vi "Telescope GUI.vi"(9 "Standalone":bool=TRUE, 10 "Init Data":variant, 11 "Telescope Name":string) -> ()   [LabVIEW 2024]
uses:
  typedefs/CC enum Operation Mode.ctl
  Telescope cluster Settings.ctl
  CC cluster Telescope Offsets.ctl
  Subsystems/SS typedef cluster Instrument Command Queue Data.ctl
  Subsystems/SS cluster Data Queue type.ctl
  Telescope.lvclass
  Telescope cluster Status.ctl
  typedefs/CC cluster RA and DEC.ctl
  Telescope enum Status.ctl
  hk-channel-class/hk-channel-class/HK Item/HK Item.lvclass
  typedefs/CC cluster Object.ctl
  typedefs/CC cluster sidereal rate.ctl
  typedefs/cc cluster muRA muDEC.ctl
  typedefs/CC cluster Alarm Data.ctl
  hk-channel-class/hk-channel-class/HK Item/HK Channel cluster Telemetry Data.ctl
  hk-channel-class/hk-channel-class/HK Item/HK Channel enum Data Type.ctl
  hk-channel-class/hk-channel-class/HK Item/HK Item.lvclass/HK Item.ctl
  hk-channel-class/hk-channel-class/HK Alarms/HK Alarm enum Status.ctl
  PRIME Telescope/PRIME Telescope.lvclass
panel:
  in  "Mode":T1
  in  "Tab Control":T2(tab)
  in  "Offsets":T3 caption="Offsets (arcSec)"
  in  "Target  DEC Deg":dbl
  in  "Target  RA Deg":dbl
  in  "Target DEC":string
  in  "Target RA":string
  out "DEC Str":string
  out "RA str":string
  out "Moving":bool
  out "Focus Position":dbl format="%.3g"
  out "DEC":dbl
  out "RA":dbl
  out "Telescope Time":timestamp
  out "Connected":bool
  in  "Target Settings":T4={"RA Proper Motion"=0.0, "DEC Proper Motion"=0.0, "Equinox"=2000.0}
  in  "Home Button":bool
  in  "Stop Button":bool
  in  "Move To":bool
  in  "Focus Home":bool
  in  "Move Focus":bool
  in  "Position":dbl format="%.3g"
  in  "Reconnect":bool
  in  "Settings Button":bool
  out "Response":string
  in  "Telescope Type":u16(ring) items=["Simulation", "PRIME"]
  out "Messages":string
  out "Cmd Sent":string
  in  "Close":bool
  out "Connect Message":string
  in  "Housekeeping Data":i32(listbox)
  # "Status"
  # "Pointing"
  # "HH:MM:SS.s"
  # "Degrees"
  # "HH:MM:SS.s"
  # "Degrees"
  # "Focus"
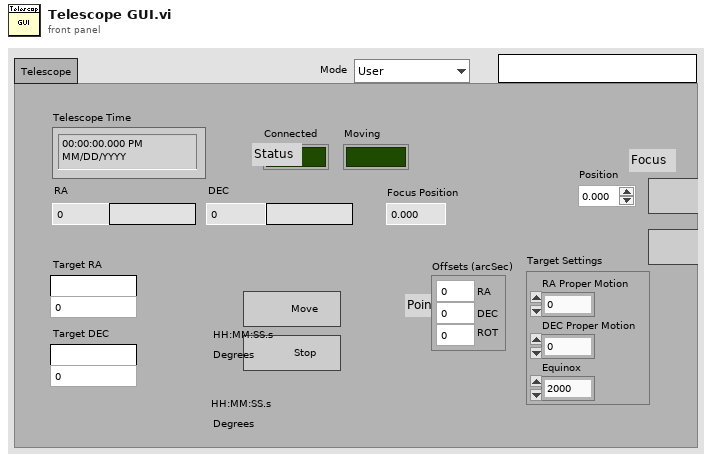
[diagram p1: front panel]
types:
  T1 = typedef "CC enum Operation Mode.ctl" = enum16{"User", "Engineering"}
  T2 = enum32{"Telescope", "Engineering", "Housekeeping"}
  T3 = typedef "CC cluster Telescope Offsets.ctl" = cluster{"RA":dbl, "DEC":dbl, "ROT":dbl}
  T4 = typedef "Telescope cluster Settings.ctl" = cluster{"RA Proper Motion":dbl, "DEC Proper Motion":dbl, "Equinox":dbl}
  T5 = typedef "SS typedef cluster Instrument Command Queue Data.ctl" = cluster{"Cmd":string, "Parameters":variant}
  T6 = typedef "Telescope.lvclass/Telescope cluster Status.ctl" = cluster{"Position":T7, "Connected":bool, "Status":T8, "Curr Time":timestamp, "Status Word":u32, "Focus Pos A":dbl, "UTC Time":timestamp, "Local Sidreal Time":dbl, "Azimuth":dbl, "Altitude":dbl, "Rotator Angle":dbl, "RA String":string, "DEC String":string, "secZ":dbl, "Focus Pos B":dbl, "Focus Pos A-B":dbl, "Rotator Offset":dbl, "Time Offset":dbl, "Dome Angle":dbl, "Dome Status Word":u32, "Dome Moving":bool}
  T7 = typedef "CC cluster RA and DEC.ctl" = cluster{"RA":dbl, "DEC":dbl}
  T8 = typedef "Telescope.lvclass/Telescope enum Status.ctl" = enum16{"Initializing", "Ready", "Moving", "Focusing", "Error"}
  T9 = typedef "CC cluster Object.ctl" = cluster{"Object":cluster{"Name":string}, "Sidereal Rate":T10, "RA and DEC":T7, "muRA muDEC Epoch":T11, "Offsets":T3}
  T10 = typedef "CC cluster sidereal rate.ctl" = cluster{"dRA":dbl, "dDEC":dbl}
  T11 = typedef "cc cluster muRA muDEC.ctl" = cluster{"muRA":dbl, "muDEC":dbl, "Epoch":dbl}
  T12 = cluster{"state":refnum<user-event>, "cmd q":refnum<queue>, "Cmd":T5, "Data Q":refnum<queue>, "error":errorcluster, "next poll":timestamp, "Telescope":refnum<class "Telescope.lvclass">, "Telescope Name":string, "poll":bool, "Telescope Status":T6, "Channel List":refnum<class "HK Item.lvclass">[], "Focus Pos":dbl, "Move Position":T9}
  T13 = typedef "CC cluster Alarm Data.ctl" = cluster{"Measured Value":dbl, "Alarm Low":dbl, "Alarm High":dbl, "Message":string, "Source":string}
  T14 = typedef "SS cluster Data Queue type.ctl" = cluster{"Source":string, "Type":string, "Data":variant}
  T15 = enum32{"Page Enabled", "Page Disabled", "Page Disabled & Grayed"}
  T16 = typedef "HK Item.lvclass/HK Channel enum Data Type.ctl" = enum16{"Floating Point", "Integer", "Enum", "String", "Waveform", "File"}
  T17 = typedef "HK Item.lvclass/HK Channel cluster Telemetry Data.ctl" = cluster{"Ch Names":string[], "Ch Values":dbl[], "Timestamp":timestamp, "Data Type":T16}
  T18 = typedef "CC cluster Device Index.ctl" = cluster{"Device Type Name":string, "Curr Device Name":string, "All Instances":string[]}
  T19 = typedef "HK Item.lvclass/HK Channel Units and Setup.ctl" = cluster{"Unit Type":string, "Units":string, "Configuration":string, "Digits":i32, "Data Type":T16, "Exponential?":bool, "Source":string}
  T20 = typedef "HK Item.lvclass/HK Alarm enum Status.ctl" = enum16{"No Alarm", "Red Low", "Red High", "Yellow Low", "Yellow High"}
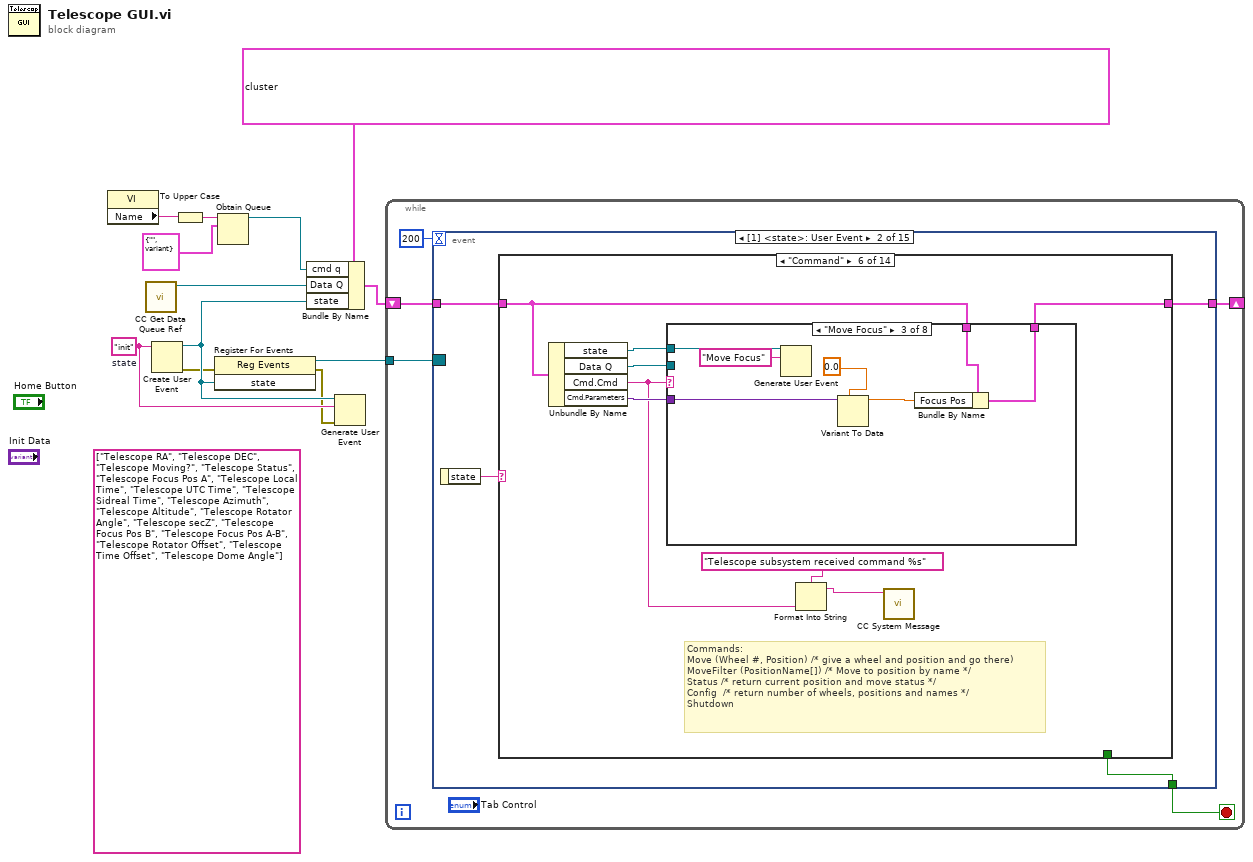
[diagram p0: block diagram]
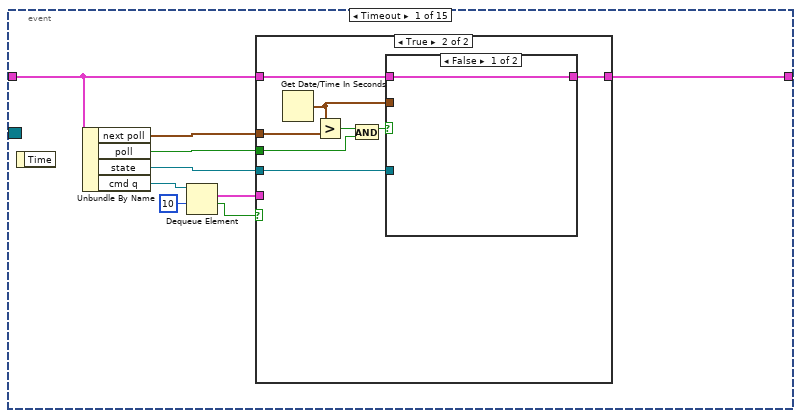
[diagram p2: hidden frame]
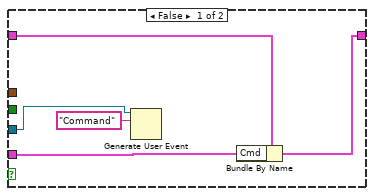
[diagram p3: hidden frame]
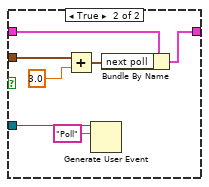
[diagram p4: hidden frame]
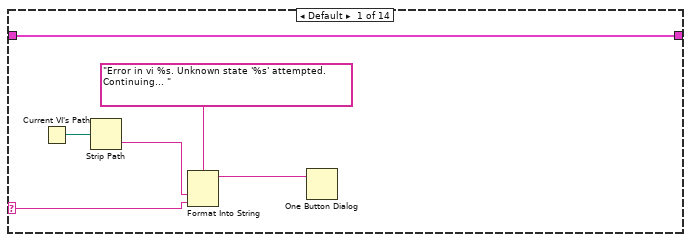
[diagram p5: hidden frame]
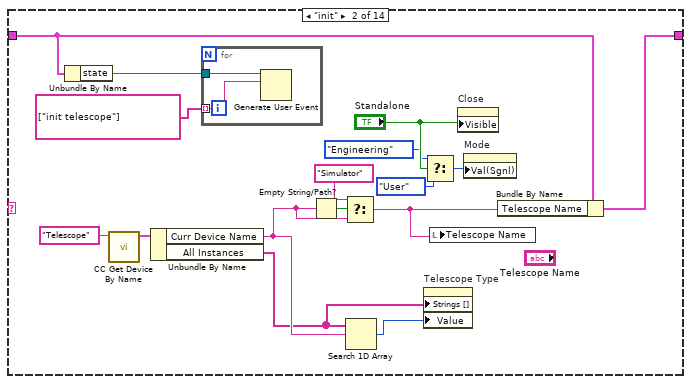
[diagram p6: hidden frame]
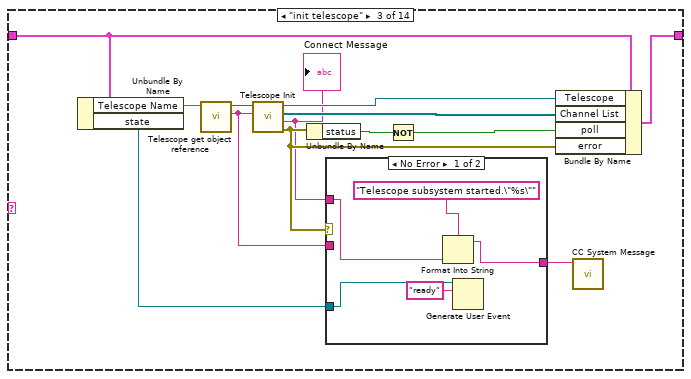
[diagram p7: hidden frame]
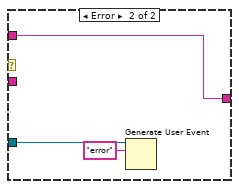
[diagram p8: hidden frame]
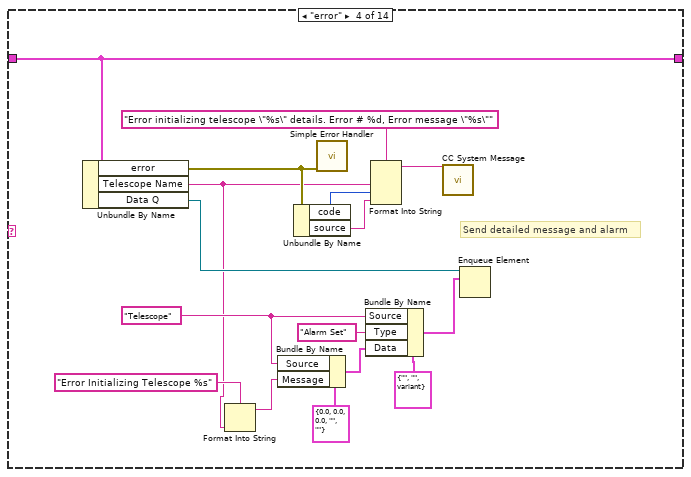
[diagram p9: hidden frame]
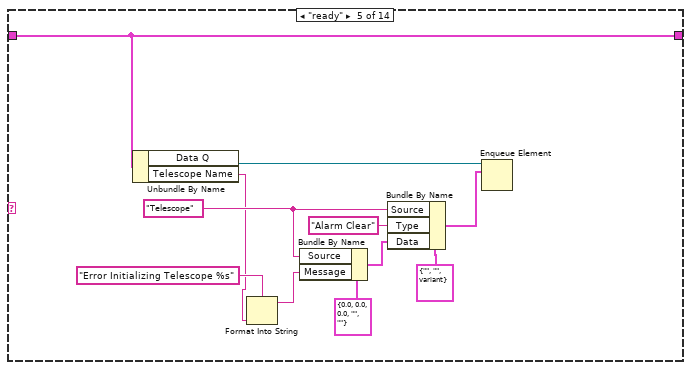
[diagram p10: hidden frame]
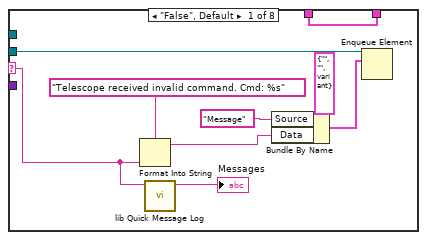
[diagram p11: hidden frame]
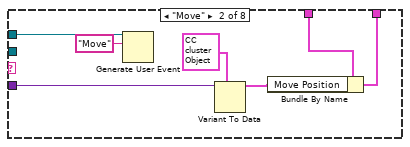
[diagram p12: hidden frame]
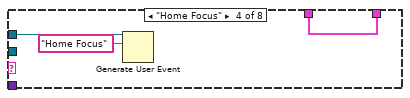
[diagram p13: hidden frame]
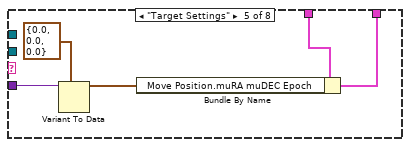
[diagram p14: hidden frame]
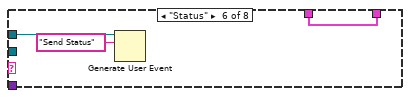
[diagram p15: hidden frame]
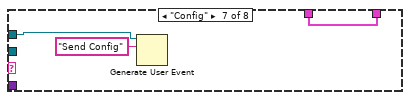
[diagram p16: hidden frame]
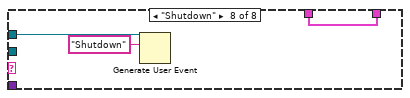
[diagram p17: hidden frame]
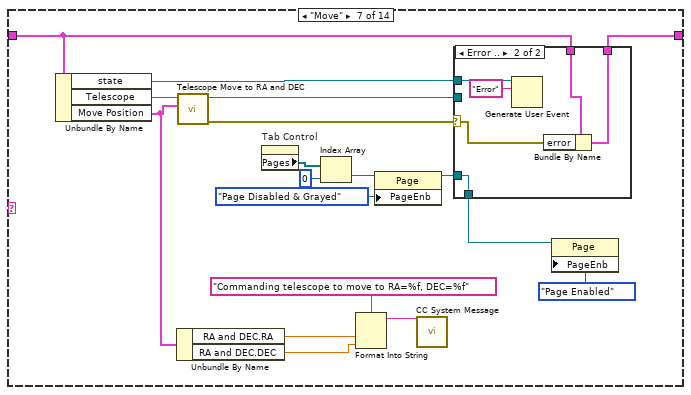
[diagram p18: hidden frame]
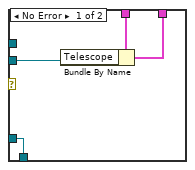
[diagram p19: hidden frame]
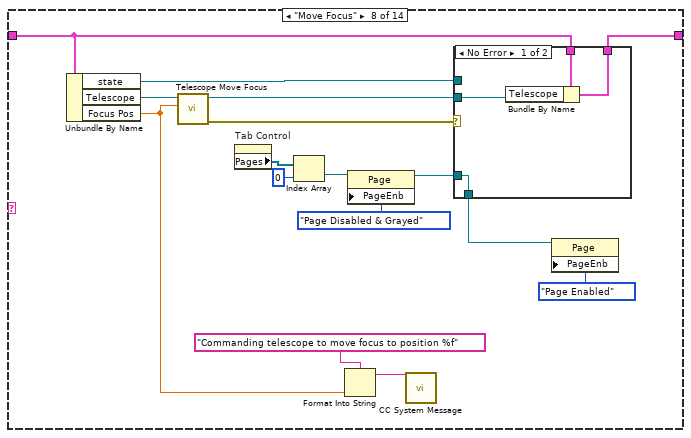
[diagram p20: hidden frame]
diagram:
  (unwired) string[] ["Telescope RA", "Telescope DEC", "Telescope Moving?", "Telescope Status", "Telescope Focus Pos A", "Telescope Local Time", "Telescope UTC Time", "Telescope Sidreal Time", "Telescope Azimuth", "Telescope Altitude", "Telescope Rotator Angle", "Telescope secZ", "Telescope Focus Pos B", "Telescope Focus Pos A-B", "Telescope Rotator Offset", "Telescope Time Offset", "Telescope Dome Angle"]
  w8 = "init"  # state
  n1 = property class="VI"() -> ("Name"=w4:string)  [unwired: 2 in, 2 out]
  n2 = call "CC Get Data Queue Ref.vi"() -> ("Data Q"=w5:refnum<queue>)  [unwired: 10 in, 1 out]
  n3 = Create User Event(user event datatype=w8) -> (user event=w10:refnum<user-event>, error out=w6:errorcluster)  [unwired: 1 in]
  n4 = To Upper Case(1:w4) -> (0:w3:string)
  n5 = register-events(error in=w6, w10) -> (reference out=w9:refnum<event-registration>, error out=w7:errorcluster)  [unwired: 1 in]
  n6 = Obtain Queue(name (unnamed)=w3, element data type=T5 {"Cmd"="", "Parameters"=variant}) -> (queue out=w1:refnum<queue>)  [unwired: 3 in, 2 out]
  n7 = Bundle By Name(cluster=T12 {"state"=refnum, "cmd q"=refnum, "Cmd"={"Cmd"="", "Parameters"=variant}, "Data Q"=refnum, "error"={"status"=FALSE, "code"=0, "source"=""}, "next poll"=timestamp(0 s since 1904-01-01), "Telescope"=refnum, "Telescope Name"="", "poll"=FALSE, "Telescope Status"={"Position"={"RA"=0.0, "DEC"=0.0}, "Connected"=FALSE, "Status"=enum."Initializing", "Curr Time"=timestamp(0 s since 1904-01-01), "Status Word"=0, "Focus Pos A"=0.0, "UTC Time"=timestamp(0 s since 1904-01-01), "Local Sidreal Time"=0.0, "Azimuth"=0.0, "Altitude"=0.0, "Rotator Angle"=0.0, "RA String"="", "DEC String"="", "secZ"=0.0, "Focus Pos B"=0.0, "Focus Pos A-B"=0.0, "Rotator Offset"=0.0, "Time Offset"=0.0, "Dome Angle"=0.0, "Dome Status Word"=0, "Dome Moving"=FALSE}, "Channel List"=[], "Focus Pos"=0.0, "Move Position"={"Object"={"Name"=""}, "Sidereal Rate"={"dRA"=0.0, "dDEC"=0.0}, "RA and DEC"={"RA"=0.0, "DEC"=0.0}, "muRA muDEC Epoch"={"muRA"=0.0, "muDEC"=0.0, "Epoch"=0.0}, "Offsets"={"RA"=0.0, "DEC"=0.0, "ROT"=0.0}}}, "cmd q"=w1, "Data Q"=w5, "state"=w10) -> (w11:T12)
  n8 = Generate User Event(user event=w10, event data cluster=w8, error in=w7) -> ()  [unwired: 1 in, 2 out]
  n9 = while {
    tunnel: w9 -> [w17]
    shift-right: [w15] -> _
    shift-left: w11 -> [w16]
    stop <- w14 stop-if-true
    n10 = event shown="[1] <state>: User Event" {
      selector: w17 -> [_ _ _ _ _ _ _ _ _ _ _ _ _ _ _]
      dyn-events: _ -> [_ _ _ _ _ _ _ _ _ _ _ _ _ _ _]
      timeout: 200 -> [_ _ _ _ _ _ _ _ _ _ _ _ _ _ _]
      tunnel: w16 -> [w21 w50 w360 w375 w378 w381 w386 w391 w394 w397 w401 w407 w414 w418 w425]
      tunnel: [w20 w49 w361 w375 w378 w381 w386 w391 w394 w397 w401 w408 w414 w418 w425] -> w15
      tunnel: [_ w48 _ _ _ _ _ _ _ _ _ _ _ _ _] -> w14
      event Timeout {
        n11 = event-data() -> ()  [unwired: 1 in, 1 out]
        n12 = Unbundle By Name(w21) -> ("next poll"=w19:timestamp, "poll"=w18:bool, "state"=w22:refnum<user-event>, "cmd q"=w26:refnum<queue>)
        n13 = Dequeue Element(queue=w26, timeout in ms (-1)=10) -> (element=w23:T5, timed out?=w24:bool)  [unwired: 1 in, 2 out]
        n14 = case shown="True" w24 {
          tunnel: w23 -> [w28 _]
          tunnel: w22 -> [w31 w36]
          tunnel: w21 -> [w29 w37]
          tunnel: [w27 w34] -> w20
          tunnel: w19 -> [_ w39]
          tunnel: w18 -> [_ w32]
          frame False {
            n15 = Generate User Event(user event=w31, event data cluster="Command" ("event data")) -> ()  [unwired: 2 in, 2 out]
            n16 = Bundle By Name(cluster=w29, "Cmd"=w28) -> (w27:T12)
          }
          frame True {
            n17 = Get Date/Time In Seconds() -> (seconds since 1Jan1904=w35:timestamp)
            n18 = Greater?(x=w35, y=w39) -> (0:w38:bool)
            n19 = And(x=w38, y=w32) -> (x .and. y?=w33:bool)
            n20 = case shown="False" w33 {
              tunnel: w37 -> [w40 w47]
              tunnel: w36 -> [_ w46]
              tunnel: w35 -> [_ w45]
              tunnel: [w40 w42] -> w34
              frame False {
              }
              frame True {
                n21 = Add(x=w45, y=3.0) -> (x+y=w43:timestamp)
                n22 = Generate User Event(user event=w46, event data cluster="Poll" ("event data")) -> ()  [unwired: 2 in, 2 out]
                n23 = Bundle By Name(cluster=w47, "next poll"=w43) -> (w42:T12)
              }
            }
          }
        }
      }
      event User Event {
        n24 = event-data() -> ("state"=w51:string)  [unwired: 1 in]
        n25 = case shown="\"Command\"" w51 {
          selector: w51 -> [w56 _ _ _ _ _ _ _ _ _ _ _ _ _]
          tunnel: w50 -> [w52 w71 w84 w112 w115 w127 w182 w208 w232 w252 w268 w292 w350 w354]
          tunnel: [w52 w72 w85 w112 w115 w128 w183 w209 w233 w252 w269 w292 w350 w354] -> w49
          tunnel: [_ _ _ _ _ _ _ _ _ _ _ _ _ TRUE] -> w48
          frame Default {
            n26 = Current VI's Path() -> (path=w55:path)
            n27 = Strip Path(path=w55) -> (name=w54:string)  [unwired: 1 out]
            n28 = Format Into String(format string="Error in vi %s. Unknown state '%s' attempted. Continuing... ", w54, w56) -> (resulting string=w53:string)  [unwired: 2 in, 1 out]
            n29 = One Button Dialog(message=w53) -> ()  [unwired: 1 in, 1 out]
          }
          frame "init" {
            n30 = Unbundle By Name(w71) -> ("state"=w70:refnum<user-event>)
            n31 = call "CC Get Device By Name.vi"("Device Type"="Telescope") -> ("Device"=w65:T18)  [unwired: 8 in, 2 out]
            n32 = Unbundle By Name(w65) -> ("Curr Device Name"=w64:string, "All Instances"=w63:string[])
            n33 = for {
              tunnel: w70 -> [w75]
              tunnel: string[] ["init telescope"] -> [w74] mode=indexing
              n34 = Generate User Event(user event=w75, event data cluster=w74) -> ()  [unwired: 2 in, 2 out]
            }
            n35 = Empty String/Path?(string/path=w64) -> (empty?=w73:bool)
            n36 = Select(t="Simulator", s=w73, f=w64) -> (s? t:f=w58:string)
            n37 = Search 1D Array(1D array=w63, element=w64) -> (index of element=w68:i32)  [unwired: 1 in]
            n38 = property on="Telescope Type" class="Ring (strict)"("Strings []"=w63, "Value"=w68) -> ()  [unwired: 2 in, 2 out]
            n39 = Select(t=CC_enum_Operation_Mode."Engineering" ("Mode"), s="Standalone", f=CC_enum_Operation_Mode."User" ("Mode")) -> (s? t:f=w59:T1)
            n40 = local write "Telescope Name"(w58) -> ()
            n41 = property on="Close" class="Bool"("Visible"="Standalone") -> ()  [unwired: 2 in, 2 out]
            n42 = property on="Mode" class="Enum (strict)"("Val(Sgnl)"=w59) -> ()  [unwired: 2 in, 2 out]
            n43 = Bundle By Name(cluster=w71, "Telescope Name"=w58) -> (w72:T12)
          }
          frame "init telescope" {
            n44 = Unbundle By Name(w84) -> ("Telescope Name"=w87:string, "state"=w78:refnum<user-event>)
            n45 = call "Telescope get object reference.vi"("Telescope Name"=w87) -> ("Telescope Name dup"=w79:string, "PRIME Telescope.lvclass"=w88:refnum<class "Telescope.lvclass">)  [unwired: 8 in, 1 out]
            n46 = call-dynamic "Telescope Init.vi"("Name"=w79, "Telescope in"=w88) -> ("error out"=w77:errorcluster, "Connect Message"=w76:string, "Channel List"=w81:refnum<class "HK Item.lvclass">[], "Telescope out"=w86:refnum<class "Telescope.lvclass">)  [unwired: 6 in]
            "Connect Message" <- w76
            n47 = Unbundle By Name(w77) -> ("status"=w83:bool)
            n48 = case shown="No Error" w77 {
              tunnel: [w93 w94] -> w80
              tunnel: w79 -> [_ _]
              tunnel: w78 -> [w90 w96]
              tunnel: w76 -> [w91 w94]
              frame No Error {
                n49 = Format Into String(format string="Telescope subsystem started.\"%s\"", w91) -> (resulting string=w93:string)  [unwired: 2 in, 1 out]
                n50 = Generate User Event(user event=w90, event data cluster="ready" ("event data")) -> ()  [unwired: 2 in, 2 out]
              }
              frame Error {
                n51 = Generate User Event(user event=w96, event data cluster="error" ("event data")) -> ()  [unwired: 2 in, 2 out]
              }
            }
            n52 = Not(x=w83) -> (.not. x?=w82:bool)
            n53 = Bundle By Name(cluster=w84, "Telescope"=w86, "Channel List"=w81, "poll"=w82, "error"=w77) -> (w85:T12)
            n54 = call "CC System Message.vi"("Message"=w80) -> ()  [unwired: 10 in, 1 out]
          }
          frame "error" {
            w107 = "Telescope" ("Source")
            # "Send detailed message and alarm"
            n55 = Unbundle By Name(w112) -> ("error"=w104:errorcluster, "Telescope Name"=w97:string, "Data Q"=w101:refnum<queue>)
            n56 = Format Into String(format string="Error Initializing Telescope %s" ("Message"), w97) -> (resulting string=w98:string)  [unwired: 2 in, 1 out]
            n57 = Bundle By Name(cluster=T13 {"Measured Value"=0.0, "Alarm Low"=0.0, "Alarm High"=0.0, "Message"="", "Source"=""} ("element"), "Source"=w107, "Message"=w98) -> (w108:T13)
            n58 = Unbundle By Name(w104) -> ("code"=w106:i32, "source"=w105:string)
            n59 = call <vilib>:"Simple Error Handler.vi"("error in (no error)"=w104) -> ()  [unwired: 4 in, 5 out]
            n60 = Bundle By Name(cluster=T14 {"Source"="", "Type"="", "Data"=variant} ("element"), "Source"=w107, "Type"="Alarm Set", "Data"=w108) -> (w100:T14)
            n61 = Format Into String(format string="Error initializing telescope \"%s\" details. Error # %d, Error message \"%s\"", w97, w106, w105) -> (resulting string=w103:string)  [unwired: 2 in, 1 out]
            n62 = call "CC System Message.vi"("Message"=w103) -> ()  [unwired: 10 in, 1 out]
            n63 = Enqueue Element(queue=w101, element=w100) -> ()  [unwired: 2 in, 3 out]
          }
          frame "ready" {
            w119 = "Telescope" ("Source")
            n64 = Unbundle By Name(w115) -> ("Data Q"=w114:refnum<queue>, "Telescope Name"=w113:string)
            n65 = Format Into String(format string="Error Initializing Telescope %s" ("Message"), w113) -> (resulting string=w116:string)  [unwired: 2 in, 1 out]
            n66 = Bundle By Name(cluster=T13 {"Measured Value"=0.0, "Alarm Low"=0.0, "Alarm High"=0.0, "Message"="", "Source"=""} ("element"), "Source"=w119, "Message"=w116) -> (w120:T13)
            n67 = Bundle By Name(cluster=T14 {"Source"="", "Type"="", "Data"=variant} ("element"), "Source"=w119, "Type"="Alarm Clear", "Data"=w120) -> (w118:T14)
            n68 = Enqueue Element(queue=w114, element=w118) -> ()  [unwired: 2 in, 3 out]
          }
          frame "Command" {
            # "Commands:\nMove (Wheel #, Position) /* give a wheel and position and go there)\nMoveFilter (PositionName[]) /* Move to position by name */\nStatus /* return current position and move status */\nConfig  /* return number of wheels, positions and names */\nShutdown"
            n69 = Unbundle By Name(w127) -> ("state"=w129:refnum<user-event>, "Data Q"=w131:refnum<queue>, "Cmd.Cmd"=w125:string, "Cmd.Parameters"=w130:variant)
            n70 = case shown="\"Move Focus\"" w125 {
              selector: w125 -> [w134 _ _ _ _ _ _ _]
              tunnel: w131 -> [w140 _ _ _ _ _ _ _]
              tunnel: w130 -> [_ w147 w154 _ w162 _ _ _]
              tunnel: w129 -> [_ w143 w150 w157 _ w165 w167 w171]
              tunnel: w127 -> [w132 w146 w153 w155 w160 w163 w166 w169]
              tunnel: [w132 w144 w151 w155 w158 w163 w166 w169] -> w128
              frame "False", Default {
                n71 = Format Into String(format string="Telescope received invalid command. Cmd: %s", w134) -> (resulting string=w136:string)  [unwired: 2 in, 1 out]
                n72 = call "lib Quick Message Log.vi"("Message"=w134) -> ("Log"=→"Messages":string)  [unwired: 9 in, 1 out]
                n73 = Bundle By Name(cluster=T14 {"Source"="", "Type"="", "Data"=variant} ("element"), "Source"="Message" ("Data Type"), "Data"=w136) -> (w135:T14)
                n74 = Enqueue Element(queue=w140, element=w135) -> ()  [unwired: 2 in, 3 out]
              }
              frame "Move" {
                n75 = Generate User Event(user event=w143, event data cluster="Move" ("event data")) -> ()  [unwired: 2 in, 2 out]
                n76 = Variant To Data(type=T9 {"Object"={"Name"=""}, "Sidereal Rate"={"dRA"=0.0, "dDEC"=0.0}, "RA and DEC"={"RA"=0.0, "DEC"=0.0}, "muRA muDEC Epoch"={"muRA"=0.0, "muDEC"=0.0, "Epoch"=0.0}, "Offsets"={"RA"=0.0, "DEC"=0.0, "ROT"=0.0}} ("Move Position"), Variant=w147) -> (data=w145:T9)  [unwired: 1 in, 1 out]
                n77 = Bundle By Name(cluster=w146, "Move Position"=w145) -> (w144:T12)
              }
              frame "Move Focus" {
                n78 = Generate User Event(user event=w150, event data cluster="Move Focus" ("event data")) -> ()  [unwired: 2 in, 2 out]
                n79 = Variant To Data(type=0.0 ("Position"), Variant=w154) -> (data=w152:dbl)  [unwired: 1 in, 1 out]
                n80 = Bundle By Name(cluster=w153, "Focus Pos"=w152) -> (w151:T12)
              }
              frame "Home Focus" {
                n81 = Generate User Event(user event=w157, event data cluster="Home Focus" ("event data")) -> ()  [unwired: 2 in, 2 out]
              }
              frame "Target Settings" {
                n82 = Variant To Data(type=T4 {"RA Proper Motion"=0.0, "DEC Proper Motion"=0.0, "Equinox"=0.0} ("Telescope Settings"), Variant=w162) -> (data=w159:T4)  [unwired: 1 in, 1 out]
                n83 = Bundle By Name(cluster=w160, "Move Position.muRA muDEC Epoch"=w159) -> (w158:T12)
              }
              frame "Status" {
                n84 = Generate User Event(user event=w165, event data cluster="Send Status" ("event data")) -> ()  [unwired: 2 in, 2 out]
              }
              frame "Config" {
                n85 = Generate User Event(user event=w167, event data cluster="Send Config" ("event data")) -> ()  [unwired: 2 in, 2 out]
              }
              frame "Shutdown" {
                n86 = Generate User Event(user event=w171, event data cluster="Shutdown" ("event data")) -> ()  [unwired: 2 in, 2 out]
              }
            }
            n87 = Format Into String(format string="Telescope subsystem received command %s", w125) -> (resulting string=w124:string)  [unwired: 2 in, 1 out]
            n88 = call "CC System Message.vi"("Message"=w124) -> ()  [unwired: 10 in, 1 out]
          }
          frame "Move" {
            n89 = Unbundle By Name(w182) -> ("state"=w184:refnum<user-event>, "Telescope"=w179:refnum<class "Telescope.lvclass">, "Move Position"=w172:T9)
            n90 = Unbundle By Name(w172) -> ("RA and DEC.RA"=w174:dbl, "RA and DEC.DEC"=w173:dbl)
            n91 = call-dynamic "Telescope Move to RA and DEC.vi"("Object out"=w172, "Telescope in"=w179) -> ("error out"=w178:errorcluster, "Telescope out"=w177:refnum<class "Telescope.lvclass">)  [unwired: 8 in]
            n92 = property on="Tab Control" class="TabCtl (strict)"() -> ("Pages"=w189:refnum<vi>[])  [unwired: 2 in, 2 out]
            n93 = Index Array(array=w189, index=0) -> (element=w187:refnum<vi>)
            n94 = Format Into String(format string="Commanding telescope to move to RA=%f, DEC=%f", w174, w173) -> (resulting string=w175:string)  [unwired: 2 in, 1 out]
            n95 = property class="Page"(reference=w187, "PageEnb"=T15."Page Disabled & Grayed" ("Page Enabled State")) -> (reference out=w181:refnum<vi>)  [unwired: 1 in, 1 out]
            n96 = call "CC System Message.vi"("Message"=w175) -> ()  [unwired: 10 in, 1 out]
            n97 = case shown="Error .." w178 {
              selector: w178 -> [_ w196]
              tunnel: w184 -> [_ w199]
              tunnel: w182 -> [w192 w197]
              tunnel: [w190 w195] -> w183
              tunnel: w181 -> [w193 w194]
              tunnel: [w193 w194] -> w180
              tunnel: w177 -> [w191 _]
              frame No Error {
                n98 = Bundle By Name(cluster=w192, "Telescope"=w191) -> (w190:T12)
              }
              frame Error {
                n99 = Generate User Event(user event=w199, event data cluster="Error" ("event data")) -> ()  [unwired: 2 in, 2 out]
                n100 = Bundle By Name(cluster=w197, "error"=w196) -> (w195:T12)
              }
            }
            n101 = property class="Page"(reference=w180, "PageEnb"=T15."Page Enabled" ("Page Enabled State")) -> ()  [unwired: 1 in, 2 out]
          }
          frame "Move Focus" {
            n102 = Unbundle By Name(w208) -> ("state"=w210:refnum<user-event>, "Telescope"=w205:refnum<class "Telescope.lvclass">, "Focus Pos"=w201:dbl)
            n103 = call-dynamic "Telescope Move Focus.vi"("Focus Pos"=w201, "Telescope in"=w205) -> ("error out"=w204:errorcluster, "Telescope out"=w203:refnum<class "Telescope.lvclass">)  [unwired: 8 in]
            n104 = property on="Tab Control" class="TabCtl (strict)"() -> ("Pages"=w215:refnum<vi>[])  [unwired: 2 in, 2 out]
            n105 = Index Array(array=w215, index=0) -> (element=w213:refnum<vi>)
            n106 = Format Into String(format string="Commanding telescope to move focus to position %f", w201) -> (resulting string=w202:string)  [unwired: 2 in, 1 out]
            n107 = property class="Page"(reference=w213, "PageEnb"=T15."Page Disabled & Grayed" ("Page Enabled State")) -> (reference out=w207:refnum<vi>)  [unwired: 1 in, 1 out]
            n108 = call "CC System Message.vi"("Message"=w202) -> ()  [unwired: 10 in, 1 out]
            n109 = case shown="No Error" w204 {
              selector: w204 -> [_ w222]
              tunnel: w210 -> [_ w225]
              tunnel: w208 -> [w218 w223]
              tunnel: [w216 w221] -> w209
              tunnel: w207 -> [w219 w220]
              tunnel: [w219 w220] -> w206
              tunnel: w203 -> [w217 _]
              frame No Error {
                n110 = Bundle By Name(cluster=w218, "Telescope"=w217) -> (w216:T12)
              }
              frame Error {
                n111 = Generate User Event(user event=w225, event data cluster="Error" ("event data")) -> ()  [unwired: 2 in, 2 out]
                n112 = Bundle By Name(cluster=w223, "error"=w222) -> (w221:T12)
              }
            }
            n113 = property class="Page"(reference=w206, "PageEnb"=T15."Page Enabled" ("Page Enabled State")) -> ()  [unwired: 1 in, 2 out]
          }
          frame "Home Focus" {
            n114 = Unbundle By Name(w232) -> ("state"=w234:refnum<user-event>, "Telescope"=w229:refnum<class "Telescope.lvclass">)
            n115 = call-dynamic "Telescope Home Focus.vi"("Telescope in"=w229) -> ("error out"=w228:errorcluster, "Telescope out"=w227:refnum<class "Telescope.lvclass">)  [unwired: 9 in]
            n116 = property on="Tab Control" class="TabCtl (strict)"() -> ("Pages"=w239:refnum<vi>[])  [unwired: 2 in, 2 out]
            n117 = Index Array(array=w239, index=0) -> (element=w237:refnum<vi>)
            n118 = property class="Page"(reference=w237, "PageEnb"=T15."Page Disabled & Grayed" ("Page Enabled State")) -> (reference out=w231:refnum<vi>)  [unwired: 1 in, 1 out]
            n119 = call "CC System Message.vi"("Message"="Commanding telescope to move focus to home position" ("format string")) -> ()  [unwired: 10 in, 1 out]
            n120 = case shown="Error .." w228 {
              selector: w228 -> [_ w246]
              tunnel: w234 -> [_ w249]
              tunnel: w232 -> [w242 w247]
              tunnel: [w240 w245] -> w233
              tunnel: w231 -> [w243 w244]
              tunnel: [w243 w244] -> w230
              tunnel: w227 -> [w241 _]
              frame No Error {
                n121 = Bundle By Name(cluster=w242, "Telescope"=w241) -> (w240:T12)
              }
              frame Error {
                n122 = Generate User Event(user event=w249, event data cluster="Error" ("event data")) -> ()  [unwired: 2 in, 2 out]
                n123 = Bundle By Name(cluster=w247, "error"=w246) -> (w245:T12)
              }
            }
            n124 = property class="Page"(reference=w230, "PageEnb"=T15."Page Enabled" ("Page Enabled State")) -> ()  [unwired: 1 in, 2 out]
          }
          frame "Stop" {
            n125 = Unbundle By Name(w252) -> ("Telescope"=w251:refnum<class "Telescope.lvclass">)
            n126 = call-dynamic "Telescope Stop.vi"("Telescope in"=w251) -> ()  [unwired: 9 in, 2 out]
            n127 = call "CC System Message.vi"("Message"="Commanding telescope to stop all motion.") -> ()  [unwired: 10 in, 1 out]
          }
          frame "Poll" {
            # "Request status from hardware"
            n128 = Unbundle By Name(w268) -> ("Telescope"=w271:refnum<class "Telescope.lvclass">, "state"=w262:refnum<user-event>)
            n129 = Generate User Event(user event=w262, event data cluster="Send Status" ("event data")) -> ()  [unwired: 2 in, 2 out]
            n130 = call-dynamic "Telescope Read Current Status.vi"("Telescope in"=w271) -> ("Raw Response"=→"Response":string, "Telescope Status"=w267:T6, "Telescope out"=w270:refnum<class "Telescope.lvclass">, "Cmd Sent"=→"Cmd Sent":string)  [unwired: 6 in, 1 out]
            n131 = Unbundle By Name(w267) -> ("Position.RA"=w257:dbl, "Position.DEC"=w256:dbl, "Curr Time"=→"Telescope Time":timestamp, "Connected"=→"Connected":bool, "Focus Pos A"=→"Focus Position":dbl, "Status"=w259:T8)
            "RA" <- w257
            "DEC" <- w256
            n132 = Bundle By Name(cluster=w268, "Telescope"=w270, "Telescope Status"=w267) -> (w269:T12)
            n133 = case shown="\"Focusing\"" w259 {
              tunnel: [FALSE FALSE TRUE TRUE FALSE] -> w258
              frame "Initializing", Default {
              }
              frame "Ready" {
              }
              frame "Moving" {
              }
              frame "Focusing" {
              }
              frame "Error" {
              }
            }
            "Moving" <- w258
            n134 = Bundle("RA"=w257, "DEC"=w256) -> (w255:cluster{"RA":dbl, "DEC":dbl})  [unwired: 1 in]
            n135 = call "PRIME Telescope Convert RA and DEC to HHMMSS.vi"("RA and DEC"=w255) -> ("Dec String"=→"DEC Str":string, "RA String"=→"RA str":string)  [unwired: 7 in, 2 out]
          }
          frame "Send Status" {
            n136 = Unbundle By Name(w292) -> ("Data Q"=w291:refnum<queue>, "Channel List"=w286:refnum<class "HK Item.lvclass">[], "Telescope Status"=w283:T6)
            n137 = for {
              tunnel: w286 -> [w296] mode=indexing
              tunnel: w283 -> [w297]
              tunnel: [w294] -> w284 mode=indexing
              tunnel: [w295] -> w285 mode=indexing
              tunnel: [w293] -> w280 mode=indexing
              n138 = call "HK Channel Read Name.vi"("HK Item in"=w296) -> ("Name"=w295:string)  [unwired: 8 in, 2 out]
              n139 = call "Read Channel Units.vi"("HK Item in"=w296) -> ("Channel Setup"=w293:T19)  [unwired: 8 in, 2 out]
              n140 = case shown="\"Telescope Dome Moving?\"" w295 {
                tunnel: w297 -> [_ w300 w302 w310 w312 w314 w316 w318 w321 w324 w326 w328 w330 w332 w334 w336 w338 w340 w342 w345]
                tunnel: [nan ("DEC") w299 w301 w308 w311 w313 w315 w317 w319 w322 w325 w327 w329 w331 w333 w335 w337 w339 w341 w343] -> w294
                frame "False", Default {
                  (unwired) HK_Alarm_enum_Status."No Alarm" ("Alarm Status")
                }
                frame "Telescope RA" {
                  n141 = Unbundle By Name(w300) -> ("Position.RA"=w299:dbl)
                }
                frame "Telescope DEC" {
                  n142 = Unbundle By Name(w302) -> ("Position.DEC"=w301:dbl)
                }
                frame "Telescope Moving?" {
                  n143 = Unbundle By Name(w310) -> ("Status"=w306:T8)
                  n144 = Equal?(x=w306, y=Telescope_enum_Status."Moving") -> (x = y?=w307:bool)
                  n145 = Equal?(x=Telescope_enum_Status."Focusing" ("y"), y=w306) -> (x = y?=w304:bool)
                  n146 = Or(x=w304, y=w307) -> (x .or. y?=w305:bool)
                  n147 = Boolean To (0,1)(Boolean=w305) -> (0, 1=w308:i16)
                }
                frame "Telescope Status" {
                  n148 = Unbundle By Name(w312) -> ("Status Word"=w311:u32)
                }
                frame "Telescope Focus Pos A" {
                  n149 = Unbundle By Name(w314) -> ("Focus Pos A"=w313:dbl)
                }
                frame "Telescope Focus Pos B" {
                  n150 = Unbundle By Name(w316) -> ("Focus Pos B"=w315:dbl)
                }
                frame "Telescope Focus Pos A-B" {
                  n151 = Unbundle By Name(w318) -> ("Focus Pos A-B"=w317:dbl)
                }
                frame "Telescope Local Time" {
                  n152 = Unbundle By Name(w321) -> ("Curr Time"=w320:timestamp)
                  n153 = To Double Precision Float(number=w320) -> (double precision float=w319:dbl)
                }
                frame "Telescope UTC Time" {
                  n154 = Unbundle By Name(w324) -> ("UTC Time"=w323:timestamp)
                  n155 = To Double Precision Float(number=w323) -> (double precision float=w322:dbl)
                }
                frame "Telescope Sidreal Time" {
                  n156 = Unbundle By Name(w326) -> ("Local Sidreal Time"=w325:dbl)
                }
                frame "Telescope Azimuth" {
                  n157 = Unbundle By Name(w328) -> ("Azimuth"=w327:dbl)
                }
                frame "Telescope Altitude" {
                  n158 = Unbundle By Name(w330) -> ("Altitude"=w329:dbl)
                }
                frame "Telescope Rotator Angle" {
                  n159 = Unbundle By Name(w332) -> ("Rotator Angle"=w331:dbl)
                }
                frame "Telescope secZ" {
                  n160 = Unbundle By Name(w334) -> ("secZ"=w333:dbl)
                }
                frame "Telescope Rotator Offset" {
                  n161 = Unbundle By Name(w336) -> ("Rotator Offset"=w335:dbl)
                }
                frame "Telescope Time Offset" {
                  n162 = Unbundle By Name(w338) -> ("Time Offset"=w337:dbl)
                }
                frame "Telescope Dome Angle" {
                  n163 = Unbundle By Name(w340) -> ("Dome Angle"=w339:dbl)
                }
                frame "Telescope Dome Status" {
                  n164 = Unbundle By Name(w342) -> ("Dome Status Word"=w341:u32)
                }
                frame "Telescope Dome Moving?" {
                  n165 = Unbundle By Name(w345) -> ("Dome Moving"=w344:bool)
                  n166 = Boolean To (0,1)(Boolean=w344) -> (0, 1=w343:i16)
                }
              }
            }
            n167 = Unbundle By Name(w283) -> ("Curr Time"=w278:timestamp)
            n168 = Bundle(cluster=T17 {"Ch Names"=[], "Ch Values"=[], "Timestamp"=timestamp(0 s since 1904-01-01), "Data Type"=enum."Floating Point"}, "Ch Names"=w285, "Ch Values"=w284, "Timestamp"=w278, "Data Type"=HK_Channel_enum_Data_Type."Floating Point") -> (w281:T17)
            n169 = call "Telescope HK Data to Table.vi"("Ch Info"=w280, "HK Data Cluster"=w281) -> ("Table"=w279:string[][])  [unwired: 9 in]
            n170 = Bundle By Name(cluster=T14 {"Source"="", "Type"="", "Data"=variant} ("element"), "Source"="Telescope", "Type"="Floating Point" ("Data Type"), "Data"=w281) -> (w288:T14)
            n171 = property on="Housekeeping Data" class="MCListbox (strict)"("ItemNames"=w279) -> ()  [unwired: 2 in, 2 out]
            n172 = Enqueue Element(queue=w291, element=w288) -> ()  [unwired: 2 in, 3 out]
          }
          frame "Reinit" {
            n173 = Unbundle By Name(w350) -> ("Telescope"=w349:refnum<class "Telescope.lvclass">, "state"=w348:refnum<user-event>)
            n174 = call-dynamic "Telescope Close.vi"("Telescope in"=w349) -> ("error out"=w346:errorcluster)  [unwired: 9 in, 1 out]
            n175 = Generate User Event(user event=w348, event data cluster="init telescope" ("event data")) -> ()  [unwired: 2 in, 2 out]
            n176 = call <vilib>:"Clear Errors.vi"("error in (no error)"=w346) -> ()  [unwired: 5 in, 2 out]
          }
          frame "Shutdown" {
            n177 = Unbundle By Name(w354) -> ("Data Q"=w353:refnum<queue>, "Telescope"=w351:refnum<class "Telescope.lvclass">)
            n178 = Release Queue(queue=w353) -> ()  [unwired: 2 in, 3 out]
            n179 = call-dynamic "Telescope Close.vi"("Telescope in"=w351) -> ()  [unwired: 9 in, 2 out]
            n180 = call "CC System Message.vi"("Message"="Telescope shutdown.") -> ()  [unwired: 10 in, 1 out]
          }
        }
      }
      event "Settings Button": Value Change {
        n181 = event-data() -> ()  [unwired: 1 in, 6 out]
        n182 = Unbundle By Name(w360) -> ("Telescope"=w363:refnum<class "Telescope.lvclass">, "Telescope Name"=w356:string, "state"=w358:refnum<user-event>)
        n183 = call-dynamic "Telescope Configure GUI.vi"("Telescope Name"=w356, "Telescope in"=w363) -> ("Telescope out"=w362:refnum<class "Telescope.lvclass">)  [unwired: 8 in, 1 out]
        n184 = Generate User Event(user event=w358, event data cluster="Reinit" ("event data")) -> ()  [unwired: 2 in, 2 out]
        n185 = Bundle By Name(cluster=w360, "Telescope"=w362) -> (w361:T12)
        n186 = call "CC System Message.vi"("Message"="Telescope settings updated.") -> ()  [unwired: 10 in, 1 out]
      }
      event "Move To": Value Change {
        n187 = event-data() -> ()  [unwired: 1 in, 1 out]
        n188 = Unbundle By Name(w375) -> ("cmd q"=w370:refnum<queue>, "Move Position"=w369:T9)
        n189 = call "PRIME Telescope Convert HHMMSS to RA and DEC Angle.vi"("Dec String"="Target DEC", "RA String"="Target RA") -> ("RA and DEC"=w367:T7)  [unwired: 7 in, 2 out]
        n190 = Bundle By Name(cluster=w369, "Object.Name"="Telescope Manual Move", "muRA muDEC Epoch"="Target Settings", "Offsets"="Offsets", "RA and DEC"=w367) -> (w368:T9)
        n191 = Bundle By Name(cluster=T5 {"Cmd"="Move", "Parameters"=variant} ("element"), "Parameters"=w368) -> (w373:T5)
        n192 = Enqueue Element(queue=w370, element=w373) -> ()  [unwired: 2 in, 3 out]
      }
      event "Target RA": Value Change {
        n193 = event-data() -> ("NewVal"=w377:string)  [unwired: 1 in]
        n194 = call "PRIME Telescope Convert HHMMSS to RA and DEC Angle.vi"("RA String"=w377) -> ("RA"=w376:dbl)  [unwired: 8 in, 2 out]
        n195 = local write "Target  RA Deg"(w376) -> ()
      }
      event "Target DEC": Value Change {
        n196 = event-data() -> ("NewVal"=w380:string)  [unwired: 1 in]
        n197 = call "PRIME Telescope Convert HHMMSS to RA and DEC Angle.vi"("Dec String"=w380) -> ("DEC"=w379:dbl)  [unwired: 8 in, 2 out]
        n198 = local write "Target  DEC Deg"(w379) -> ()
      }
      event "Target  RA Deg": Value Change {
        n199 = event-data() -> ()  [unwired: 1 in, 6 out]
        n200 = Bundle By Name(cluster=T7 {"RA"=0.0, "DEC"=0.0} ("RA and DEC"), "RA"="Target  RA Deg") -> (w383:T7)
        n201 = call "PRIME Telescope Convert RA and DEC to HHMMSS.vi"("RA and DEC"=w383) -> ("RA String"=w382:string)  [unwired: 7 in, 3 out]
        n202 = local write "Target RA"(w382) -> ()
      }
      event "Target  DEC Deg": Value Change {
        n203 = event-data() -> ()  [unwired: 1 in, 6 out]
        n204 = Bundle By Name(cluster=T7 {"RA"=0.0, "DEC"=0.0} ("RA and DEC"), "DEC"="Target  DEC Deg") -> (w389:T7)
        n205 = call "PRIME Telescope Convert RA and DEC to HHMMSS.vi"("RA and DEC"=w389) -> ("Dec String"=w387:string)  [unwired: 7 in, 3 out]
        n206 = local write "Target DEC"(w387) -> ()
      }
      event "Stop Button": Value Change {
        n207 = event-data() -> ()  [unwired: 1 in, 6 out]
        n208 = Unbundle By Name(w394) -> ("state"=w393:refnum<user-event>)
        n209 = Generate User Event(user event=w393, event data cluster="Stop" ("event data")) -> ()  [unwired: 2 in, 2 out]
      }
      event "Move Focus": Value Change {
        n210 = event-data() -> ()  [unwired: 1 in, 6 out]
        n211 = Unbundle By Name(w397) -> ("cmd q"=w399:refnum<queue>)
        n212 = Bundle By Name(cluster=T5 {"Cmd"="Move Focus", "Parameters"=variant} ("element"), "Parameters"="Position") -> (w395:T5)
        n213 = Enqueue Element(queue=w399, element=w395) -> ()  [unwired: 2 in, 3 out]
      }
      event "Focus Home": Value Change {
        n214 = event-data() -> ()  [unwired: 1 in, 6 out]
        n215 = Unbundle By Name(w401) -> ("cmd q"=w402:refnum<queue>)
        n216 = Enqueue Element(queue=w402, element=T5 {"Cmd"="Home Focus", "Parameters"=variant}) -> ()  [unwired: 2 in, 3 out]
      }
      event "Telescope Type": Value Change {
        n217 = event-data() -> ("CtlRef"=w411:refnum<vi>)  [unwired: 1 in, 5 out]
        n218 = property class="Ring (strict)"(reference=w411) -> ("Strings []"=w410:string[])  [unwired: 1 in, 2 out]
        n219 = Unbundle By Name(w407) -> ("state"=w406:refnum<user-event>)
        n220 = Generate User Event(user event=w406, event data cluster="Reinit" ("event data")) -> ()  [unwired: 2 in, 2 out]
        n221 = Index Array(array=w410, index="Telescope Type") -> (element=w403:string)
        n222 = call "CC Set Device By Name.vi"("Device Name"=w403, "Device Type"="Telescope") -> ()  [unwired: 8 in, 2 out]
        n223 = Bundle By Name(cluster=w407, "Telescope Name"=w403) -> (w408:T12)
      }
      event "Reconnect": Value Change {
        n224 = event-data() -> ()  [unwired: 1 in, 6 out]
        n225 = Unbundle By Name(w414) -> ("state"=w413:refnum<user-event>)
        n226 = Generate User Event(user event=w413, event data cluster="Reinit" ("event data")) -> ()  [unwired: 2 in, 2 out]
      }
      event Value Change {
        n227 = event-data() -> ()  [unwired: 1 in, 6 out]
        n228 = case shown="\"User\", Default" "Mode" {
          tunnel: [bool[] [TRUE, FALSE, FALSE] bool[] [TRUE, TRUE, TRUE]] -> w415
          frame "User", Default {
          }
          frame "Engineering" {
          }
        }
        n229 = property on="Tab Control" class="TabCtl (strict)"() -> ("Pages"=w416:refnum<vi>[])  [unwired: 2 in, 2 out]
        n230 = for {
          tunnel: w416 -> [w420] mode=indexing
          tunnel: w415 -> [w419] mode=indexing
          n231 = property class="Page"(reference=w420, "PageVis"=w419) -> ()  [unwired: 1 in, 2 out]
        }
      }
      event "Close": Value Change {
        n232 = event-data() -> ()  [unwired: 1 in, 2 out]
        n233 = Unbundle By Name(w425) -> ("state"=w424:refnum<user-event>)
        n234 = Generate User Event(user event=w424, event data cluster="Shutdown" ("event data")) -> ()  [unwired: 2 in, 2 out]
      }
    }
  }
